vi "CalculateVelAtPoints.vi"(8 "MaxVels":dbl[](array[numeric]), 9 "MaxVel":dbl, 10 "MaxAccel":dbl, 11 "DistancesToEnd":dbl[](array[numeric])) -> (3 "Vel":dbl[](array[numeric]))   [LabVIEW 2017]
panel:
  out "Waveform Graph":dbl[](graph)
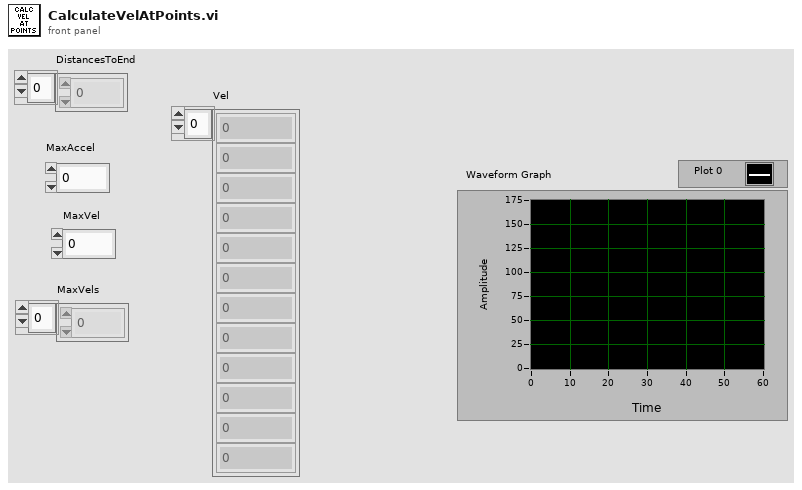
[diagram p1: front panel]
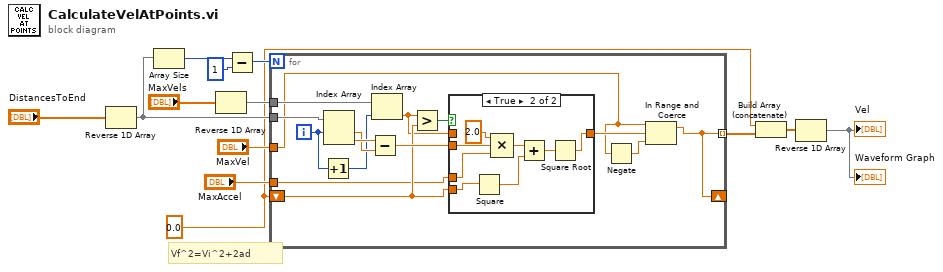
[diagram p0: block diagram]
diagram:
  w3 = 0.0 ("MaxAccel")
  # "Vf^2=Vi^2+2ad"
  n1 = Reverse 1D Array(array="DistancesToEnd") -> (reversed array=w6:dbl[])
  n2 = Array Size(array=w6) -> (size(s)=w13:i32)
  n3 = Reverse 1D Array(array="MaxVels") -> (reversed array=w5:dbl[])
  n4 = Subtract(x=w13, y=1) -> (x-y=w11:i32)
  n5 = for {
    N: w11 -> [_]
    tunnel: w6 -> [w28]
    shift-right: [w17] -> _
    shift-left: w3 -> [w20]
    tunnel: "MaxAccel" -> [w19]
    tunnel: "MaxVel" -> [w14]
    tunnel: w5 -> [w25]
    tunnel: [w17] -> w4 mode=indexing
    i -> [w24]
    n6 = Increment(x=w24) -> (x+1=w23:i32)
    n7 = Index Array(array=w28, index #1=w24) -> (element #1=w26:dbl, element #2=w27:dbl)  [unwired: 1 in]
    n8 = Subtract(x=w27, y=w26) -> (x-y=w21:dbl)
    n9 = Index Array(array=w25, index=w23) -> (element=w15:dbl)
    n10 = Greater?(x=w15, y=w20) -> (0:w22:bool)
    n11 = case shown="True" w22 {
      tunnel: w21 -> [_ w35]
      tunnel: [w29 w30] -> w18
      tunnel: w20 -> [_ w37]
      tunnel: w15 -> [w29 _]
      tunnel: w19 -> [_ w34]
      frame False {
      }
      frame True {
        n12 = Square(x=w37) -> (x^2=w33:dbl)
        n13 = Compound Arithmetic op=MULTIPLY(2.0 ("value"), w35, w34) -> (w32:dbl)
        n14 = Add(x=w32, y=w33) -> (x+y=w31:dbl)
        n15 = Square Root(x=w31) -> (sqrt(x)=w30:dbl)
      }
    }
    n16 = Negate(x=w14) -> (-x=w16:dbl)
    n17 = In Range and Coerce(upper limit=w14, x=w18, lower limit=w16) -> (coerced(x)=w17:dbl)  [unwired: 1 out]
  }
  n18 = Build Array (concatenate)(w3, w4) -> (w2:dbl[])
  n19 = Reverse 1D Array(array=w2) -> (reversed array=→"Vel" →"Waveform Graph":dbl[])
